vi "4_5_b.vi"() -> ()   [LabVIEW 2020]
uses:
  <vilib>/numeric/Random Number (Range) U64.vi
  <vilib>/numeric/sub_Random U32.vi
panel:
  out "x-y":u32
  out "Array":u64[](array[numeric])
  in  "Numeric":i32
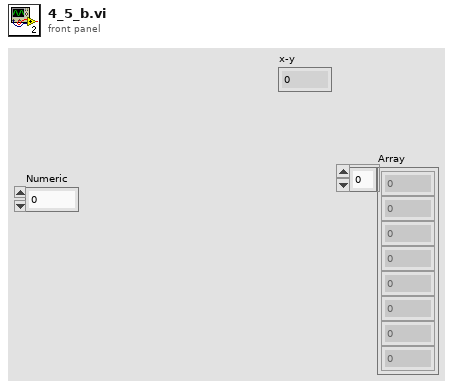
[diagram p1: front panel]
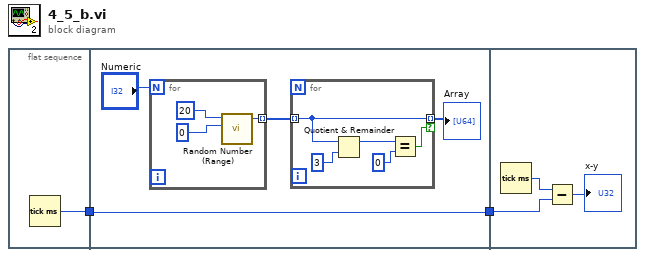
[diagram p0: block diagram]
diagram:
  n1 = flat-sequence {
    tunnel: [w3] -> w2
    tunnel: w2 -> [w6]
    tunnel: [w6] -> w1
    tunnel: w1 -> [w17]
    frame #0 {
      n2 = Tick Count (ms)() -> (millisecond timer value=w3:u32)
    }
    frame #1 {
      n3 = for {
        N: "Numeric" -> [_]
        tunnel: [w13] -> w4 mode=indexing
        n4 = call-poly <vilib>:"Random Number (Range).vi"("lower bound (0)"=u64 0, "upper bound (100)"=u64 20) -> ("number"=w13:u64)  [unwired: 9 in]
      }
      n5 = for {
        tunnel: w4 -> [w9] mode=indexing
        tunnel: [w9] -> w5 mode=indexing if=w8
        n6 = Quotient & Remainder(x=w9, y=u64 3) -> (x-y*floor(x/y)=w11:u64)  [unwired: 1 out]
        n7 = Equal?(x=w11, y=u64 0) -> (x = y?=w8:bool)
      }
      "Array" <- w5
    }
    frame #2 {
      n8 = Tick Count (ms)() -> (millisecond timer value=w18:u32)
      n9 = Subtract(x=w18, y=w17) -> (x-y=→"x-y":u32)
    }
  }
